vi "Check for Invalid Plugins.vi"() -> ()   [LabVIEW 2020, in "RxnRover.lvlib"]
uses:
  RxnRover.lvlib
  Plugin Servers/Controller/Controller Type.ctl
  Plugin Servers/Controller/Generic Plugin.lvclass
  Plugin Types.ctl
  Plugin Manager.lvlib
  Config Error.ctl
  Plugin Details.ctl
panel:
  out "error out":errorcluster
  in  "error in (no error)":errorcluster
  out "Invalid Plugins":T1[](array[typedef])
  out "Valid plugins":T1[](array[typedef])
  in  "Full Plugin Array":T1[](array[typedef])
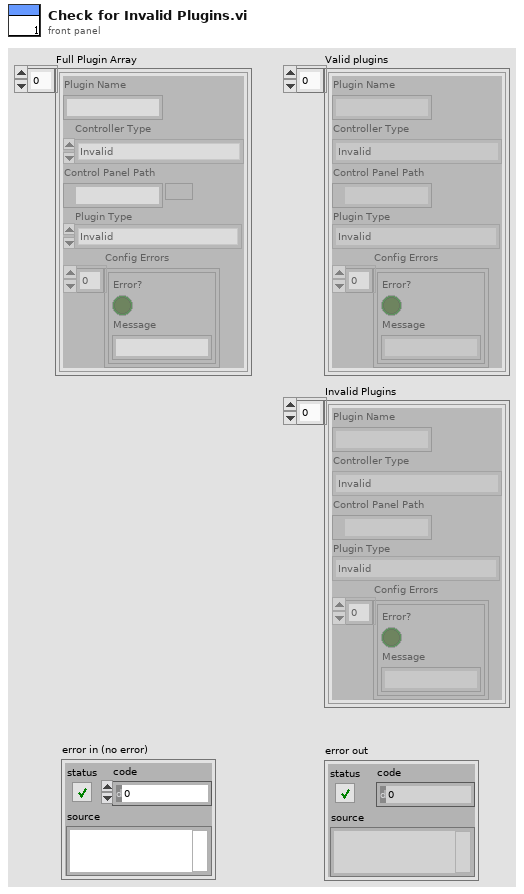
[diagram p1: front panel]
types:
  T1 = typedef "RxnRover.lvlib/Plugin Manager.lvlib/Plugin Details.ctl" = cluster{"Plugin Name":string, "Controller Type":T2, "Control Panel Path":path, "Plugin Type":T3, "Config Errors":T4[]}
  T2 = typedef "RxnRover.lvlib/Generic Plugin.lvclass/Controller Type.ctl" = enum16{"Invalid", "Temperature Controller", "Pump Controller", "Syringe Pump", "Generic Optimizer", "LC Parser"}
  T3 = typedef "RxnRover.lvlib/Plugin Manager.lvlib/Plugin Types.ctl" = enum16{"Invalid", "Optimizer", "Analyzer", "Hardware"}
  T4 = typedef "RxnRover.lvlib/Plugin Manager.lvlib/Config Error.ctl" = cluster{"Error?":bool, "Message":string}
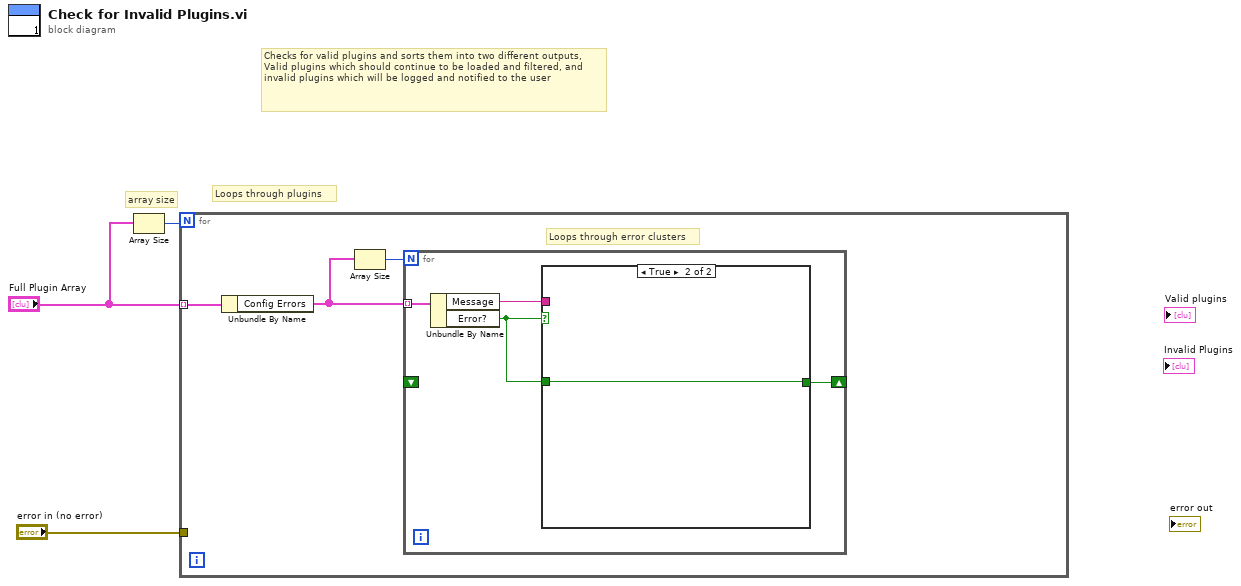
[diagram p0: block diagram]
diagram:
  # "array size"
  # "Loops through plugins"
  # "Checks for valid plugins and sorts them into two different outputs, Valid plugins which should continue to be loaded and filtered, and invalid plugins which will be logged and notified to the user"
  n1 = Array Size(array="Full Plugin Array") -> (size(s)=w3:i32)
  n2 = for {
    N: w3 -> [_]
    tunnel: "Full Plugin Array" -> [w6] mode=indexing
    tunnel: "error in (no error)" -> [_]
    # "Loops through error clusters"
    n3 = Unbundle By Name(w6) -> ("Config Errors"=w4:T4[])
    n4 = Array Size(array=w4) -> (size(s)=w5:i32)
    n5 = for {
      N: w5 -> [_]
      tunnel: w4 -> [w10] mode=indexing
      shift-right: [w7] -> _
      shift-left: _ -> [_]
      n6 = Unbundle By Name(w10) -> ("Message"=w9:string, "Error?"=w8:bool)
      n7 = case shown="True" w8 {
        tunnel: w9 -> [_ _]
        tunnel: [_ w11] -> w7
        tunnel: w8 -> [_ w11]
        frame False {
        }
        frame True {
        }
      }
    }
  }
